vi "Create Error Codes.vi"(8 "error in (no error)":errorcluster, 10 "Error Codes":cluster{"Code":i32, "String":string}[](array[cluster]), 11 "Message Channels Section in":T1 format="%.0x") -> (0 "error out":errorcluster, 3 "Message Channels Section out":T1 format="%.0x")   [LabVIEW 2020, in "Instrument Addon Scripting API.lvlib"]
uses:
  Instrument Addon Scripting API.lvlib
  <vilib>/NI VeriStand/Custom Device API/Custom Device Item Ref.ctl
  <vilib>/NI VeriStand/Custom Device API/Custom Device Channel.ctl
  <vilib>/NI VeriStand/Custom Device API/Custom Device Channel Type.ctl
  NationalInstruments.VeriStand.SystemDefinitionAPI
  NationalInstruments.VeriStand.SystemStorage
  Shared Directory/Constants.vi
  Shared Directory/Instrument Addon Shared.lvlib
  <vilib>/NI VeriStand/Custom Device API/Custom Device API.lvlib
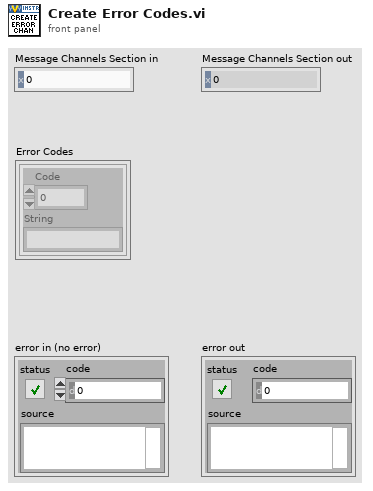
[diagram p1: front panel]
types:
  T1 = typedef "Custom Device API.lvlib/Custom Device Item Ref.ctl" = u64
  T2 = typedef "Custom Device API.lvlib/Custom Device Channel.ctl" = cluster{"Type":T3, "Units":string, "Default Value":dbl, "Faultable":bool, "Scalable":bool}
  T3 = typedef "Custom Device API.lvlib/Custom Device Channel Type.ctl" = enum16{"Input", "Output"}
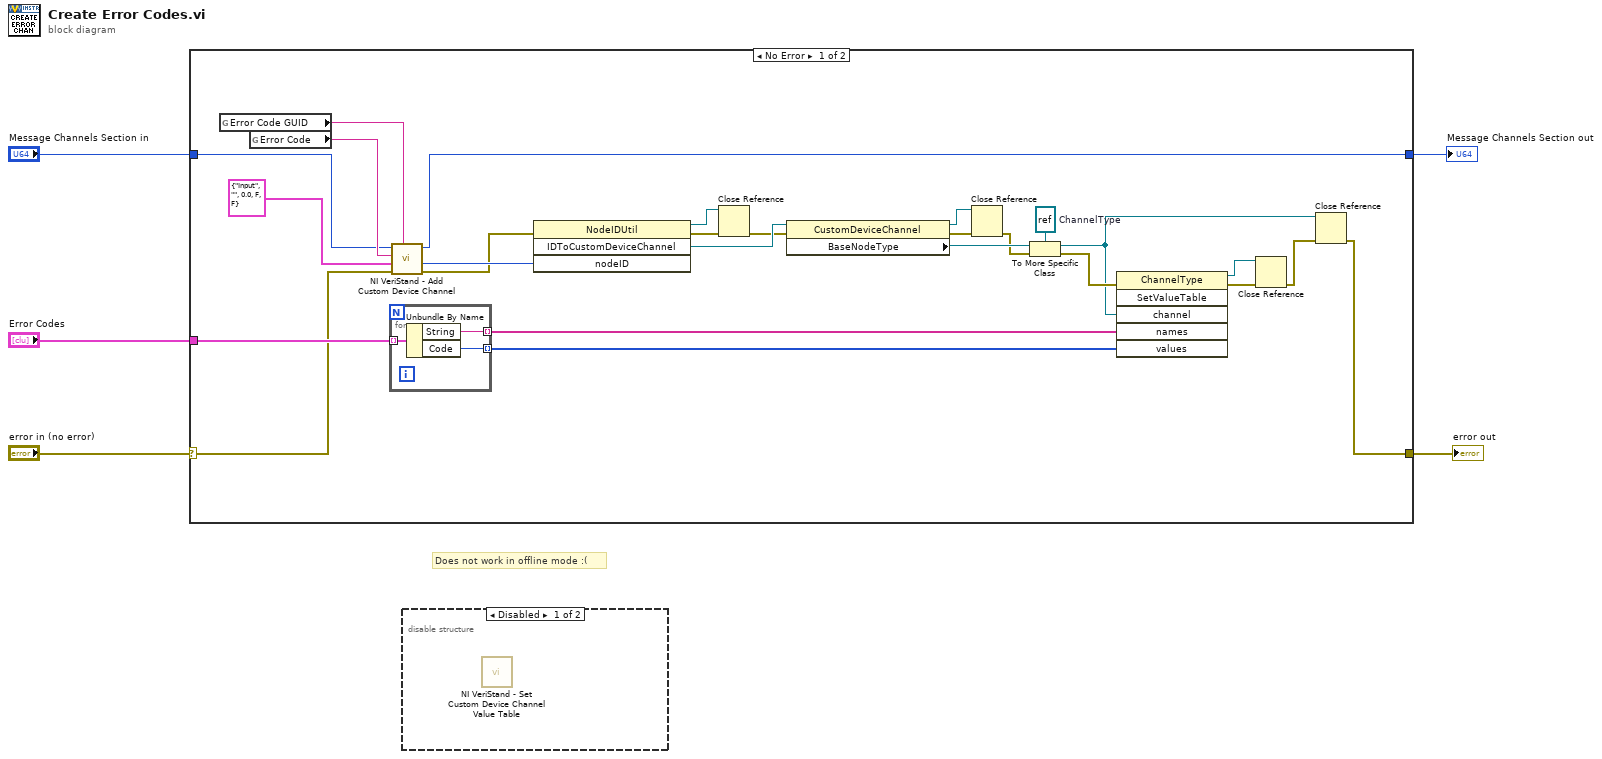
[diagram p0: block diagram]
diagram:
  # "Does not work in offline mode :("
  n1 = case shown="No Error" "error in (no error)" {
    selector: "error in (no error)" -> [w6 w35]
    tunnel: "Error Codes" -> [w30 _]
    tunnel: "Message Channels Section in" -> [w27 w36]
    tunnel: [w8 w35] -> w3
    tunnel: [w7 w36] -> w2
    frame No Error {
      w24 = refnum<k24> refnum  # ChannelType
      n2 = global read "Constants.vi" "Error Code GUID"() -> (w28:string)
      n3 = global read "Constants.vi" "Error Code"() -> (w29:string)
      n4 = for {
        tunnel: w30 -> [w34] mode=indexing
        tunnel: [w33] -> w21 mode=indexing
        tunnel: [w32] -> w20 mode=indexing
        n5 = Unbundle By Name(w34) -> ("String"=w33:string, "Code"=w32:i32)
      }
      n6 = call <vilib>:"NI VeriStand - Add Custom Device Channel.vi"("GUID (Default Channel)"=w28, "error in (no error)"=w6, "Channel"=T2 {"Type"=enum."Input", "Units"="", "Default Value"=0.0, "Faultable"=FALSE, "Scalable"=FALSE}, "Channel Name"=w29, "Parent Ref in"=w27) -> ("error out"=w19:errorcluster, "Channel Ref"=w23:T1, "Parent Ref out"=w7:T1)  [unwired: 3 in, 1 out]
      n7 = invoke class="NodeIDUtil" method="IDToCustomDeviceChannel"(error in=w19, "nodeID"=w23) -> (reference out=w17:refnum<k24>, error out=w18:errorcluster, "IDToCustomDeviceChannel"=w26:refnum<k24>)  [unwired: 2 in, 1 out]
      n8 = Close Reference(reference=w17, error in (no error)=w18) -> (error out=w16:errorcluster)
      n9 = property class="CustomDeviceChannel"(reference=w26, error in=w16) -> (reference out=w10:refnum<k24>, error out=w11:errorcluster, "BaseNodeType"=w22:refnum<k24>)
      n10 = Close Reference(reference=w10, error in (no error)=w11) -> (error out=w9:errorcluster)
      n11 = To More Specific Class(target class=w24, reference=w22, error in=w9) -> (specific class reference=w12:refnum<k24>, error out=w25:errorcluster)
      n12 = invoke class="ChannelType" method="SetValueTable"(error in=w25, "channel"=w12, "names"=w21, "values"=w20) -> (reference out=w14:refnum<k24>, error out=w15:errorcluster)  [unwired: 2 in, 4 out]
      n13 = Close Reference(reference=w14, error in (no error)=w15) -> (error out=w13:errorcluster)
      n14 = Close Reference(reference=w12, error in (no error)=w13) -> (error out=w8:errorcluster)
    }
    frame Error {
    }
  }
  "error out" <- w3
  "Message Channels Section out" <- w2
  n15 = disable-structure shown="Disabled" {
    frame Disabled {
      n16 = call <vilib>:"NI VeriStand - Set Custom Device Channel Value Table.vi"() -> ()  [unwired: 10 in, 2 out]
    }
    frame Enabled {
    }
  }
